vi "Sound-InitDevice.vi"(0 "Error Message":string="Problemas al Inicializar el Sonido", 1 "Sound Parameters":T2={"device ID"=0, "sound format"={"sample rate (S/s)"=44000.0, "number of channels"=2, "bits per sample"=16}, "time (ms)"=200.0}) -> (2 "Sound Device OUT":T4 {"task ID" format="%.0x"}, 3 "# samples":u32, 4 "Inizializo?":bool, 5 "task ID":T3 format="%.0x")   [LabVIEW 2010]
uses:
  <vilib>/sound2/lvsound2.llb/Sound Output Task ID.ctl
  <vilib>/sound2/lvsound2.llb/Sound Data Format.ctl
  <vilib>/sound2/lvsound2.llb/Sampling Mode.ctl
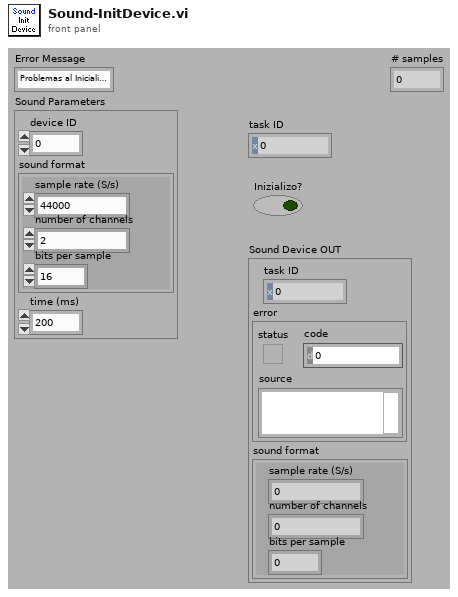
[diagram p1: front panel]
types:
  T1 = typedef "Sound Data Format.ctl" = cluster{"sample rate (S/s)":dbl, "number of channels":i32, "bits per sample":i32}
  T2 = cluster{"device ID":u32, "sound format":T1, "time (ms)":dbl}
  T3 = typedef "Sound Output Task ID.ctl" = u32
  T4 = cluster{"task ID":T3, "error":errorcluster, "sound format":T1}
  T5 = typedef "Sampling Mode.ctl" = i32
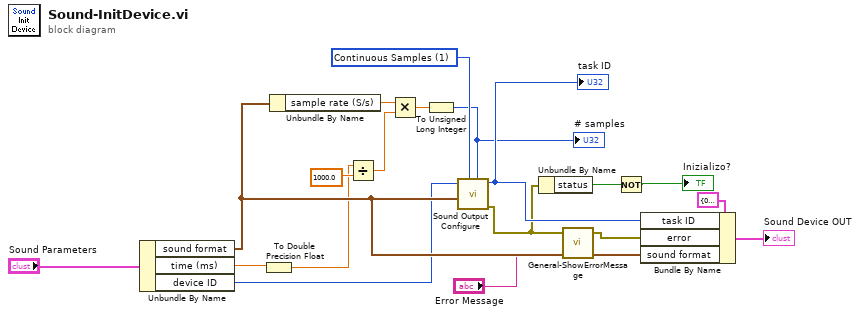
[diagram p0: block diagram]
diagram:
  w13 = T5 1 items=["Finite Samples", "Continuous Samples"] ("sample mode")
  n1 = Unbundle By Name("Sound Parameters") -> ("sound format"=w18:T1, "time (ms)"=w2:dbl, "device ID"=w14:u32)
  n2 = To Double Precision Float(number=w2) -> (double precision float=w1:dbl)
  n3 = Unbundle By Name(w18) -> ("sample rate (S/s)"=w10:dbl)
  n4 = Divide(x=w1, y=sgl 1000.0) -> (x/y=w9:dbl)
  n5 = Multiply(x=w10, y=w9) -> (x*y=w12:dbl)
  n6 = To Unsigned Long Integer(number=w12) -> (unsigned 32bit integer=w8:u32)
  "# samples" <- w8
  n7 = call <vilib>:"Sound Output Configure.vi"("number of samples/ch"=w8, "sample mode"=w13, "sound format"=w18, "device ID"=w14) -> ("error out"=w4:errorcluster, "task ID"=w17:T3)  [unwired: 6 in]
  "task ID" <- w17
  n8 = Unbundle By Name(w4) -> ("status"=w3:bool)
  n9 = call "General-ShowErrorMessage.vi"("message"="Error Message", "Error IN"=w4) -> ("Error OUT"=w5:errorcluster)  [unwired: 3 in]
  n10 = Not(x=w3) -> (.not. x?=→"Inizializo?":bool)
  n11 = Bundle By Name(cluster=T4 {"task ID"=0, "error"={"status"=FALSE, "code"=0, "source"=""}, "sound format"={"sample rate (S/s)"=0.0, "number of channels"=0, "bits per sample"=0}} ("Sound Device IN"), "task ID"=w17, "error"=w5, "sound format"=w18) -> (→"Sound Device OUT":T4)
